vi "Teleop.vi"(10 "Match Info":T1={"Autonomous Elapsed Seconds"=0.0, "TeleOp Elapsed Seconds"=0.0, "Disabled Elapsed Seconds"=0.0, "Visited Autonomous"=FALSE, "Visited TeleOp"=FALSE, "Visited Disabled"=FALSE, "Autonomous Settings"={"Autonomous Style"=enum."Independent", "VI Refnum"=refnum}}, 11 "Call Context":T2) -> ()   [LabVIEW 2015]
doc: "This VI is called for each TeleOp packet received from the DS where the robot is not disabled. It is often used to read from the joysticks and update I/O or to update setpoints for timed control loops. It should complete and return within 20 milliseconds or it may miss DS packets."
uses:
  <vilib>/Rock Robotics/WPI/DriverStation/WPI_DriverStationDerivedRobotMode.ctl
  <vilib>/Rock Robotics/WPI/DriverStation/WPI_DriverStationMatch Info.ctl
  <vilib>/Rock Robotics/WPI/Utilities/WPI_GetSetVariantRefNum.vi
  <vilib>/Rock Robotics/Network Tables/NT Read Boolean.vi
  <vilib>/Rock Robotics/Network Tables/NT Read Number.vi
  Robot Global Data.vi
  <vilib>/Rock Robotics/Network Tables/NT Write Numeric Array.vi
panel:
  out "Sample Slider 0":dbl(slide) scale=0.0..5.0
  out "Sample Boolean 1":bool
  out "Sample Boolean 0":bool
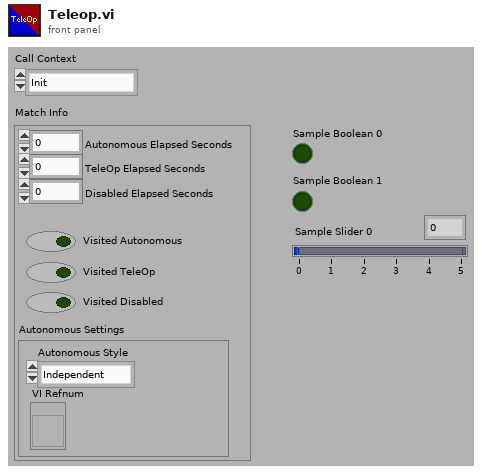
[diagram p1: front panel]
types:
  T1 = typedef "WPI_DriverStationMatch Info.ctl" = cluster{"Autonomous Elapsed Seconds":dbl, "TeleOp Elapsed Seconds":dbl, "Disabled Elapsed Seconds":dbl, "Visited Autonomous":bool, "Visited TeleOp":bool, "Visited Disabled":bool, "Autonomous Settings":cluster{"Autonomous Style":enum16{"Iterative", "Independent"}, "VI Refnum":refnum<vi>}}
  T2 = typedef "WPI_DriverStationDerivedRobotMode.ctl" = enum16{"Init", "Execute", "Stop"}
  T3 = typedef "WPI_JoystickDevRef.ctl" = cluster{"Device":T4}
  T4 = typedef "WPI_JoystickDeviceEnum.ctl" = enum16{"USB 0", "USB 1", "USB 2", "USB 3", "USB 4", "USB 5"}
  T5 = typedef "WPI_RobotDriveDevRef.ctl" = cluster{"DevStatus":errorcluster, "Motors[]":T6[], "Square Inputs":bool, "Max Output":dbl}
  T6 = typedef "WPI_MotorControlDeviceRef.ctl" = cluster{"DeviceStatus":errorcluster, "Type":T7, "PWM":cluster{"PWM Channel":T8, "DeadBand":T9}, "CAN":cluster{"Device Number":u8, "Control Mode":T10, "Semaphore":T11, "Max Vout":dbl, "TalonSRX Control Mode":T12}, "Invert":bool}
  T7 = typedef "WPI_MotorControlType.ctl" = enum16{"PWM", "CAN", "CANTalonSRX"}
  T8 = typedef "FPGA_DIOPWMChannel.ctl" = enum8{"PWM 0", "PWM 1", "PWM 2", "PWM 3", "PWM 4", "PWM 5", "PWM 6", "PWM 7", "PWM 8", "PWM 9", "PWM MXP 0", "PWM MXP 1", "PWM MXP 2", "PWM MXP 3", "PWM MXP 4", "PWM MXP 5", "PWM MXP 6", "PWM MXP 7", "PWM MXP 8", "PWM MXP 9", "Invalid"}
  T9 = typedef "WPI_PWMDeadband.ctl" = cluster{"Name":string, "maxPositivePwm":i32, "minPositivePwm":i32, "centerPwm":i32, "maxNegativePwm":i32, "minNegativePwm":i32, "angularRange":u16}
  T10 = typedef "WPI_CANJaguar_ControlMode.ctl" = enum8{"Percent VBus", "Current", "Speed", "Position", "Voltage"}
  T11 = typedef "Semaphore RefNum" = refnum<k1>
  T12 = typedef "WPI_CANTalonSRX_APIControlMode.ctl" = enum8{"Percent VBus", "Speed", "Position", "Slave", "Unchanged / Invalid", "Voltage Compensation", "Current", "Motion Profile"}
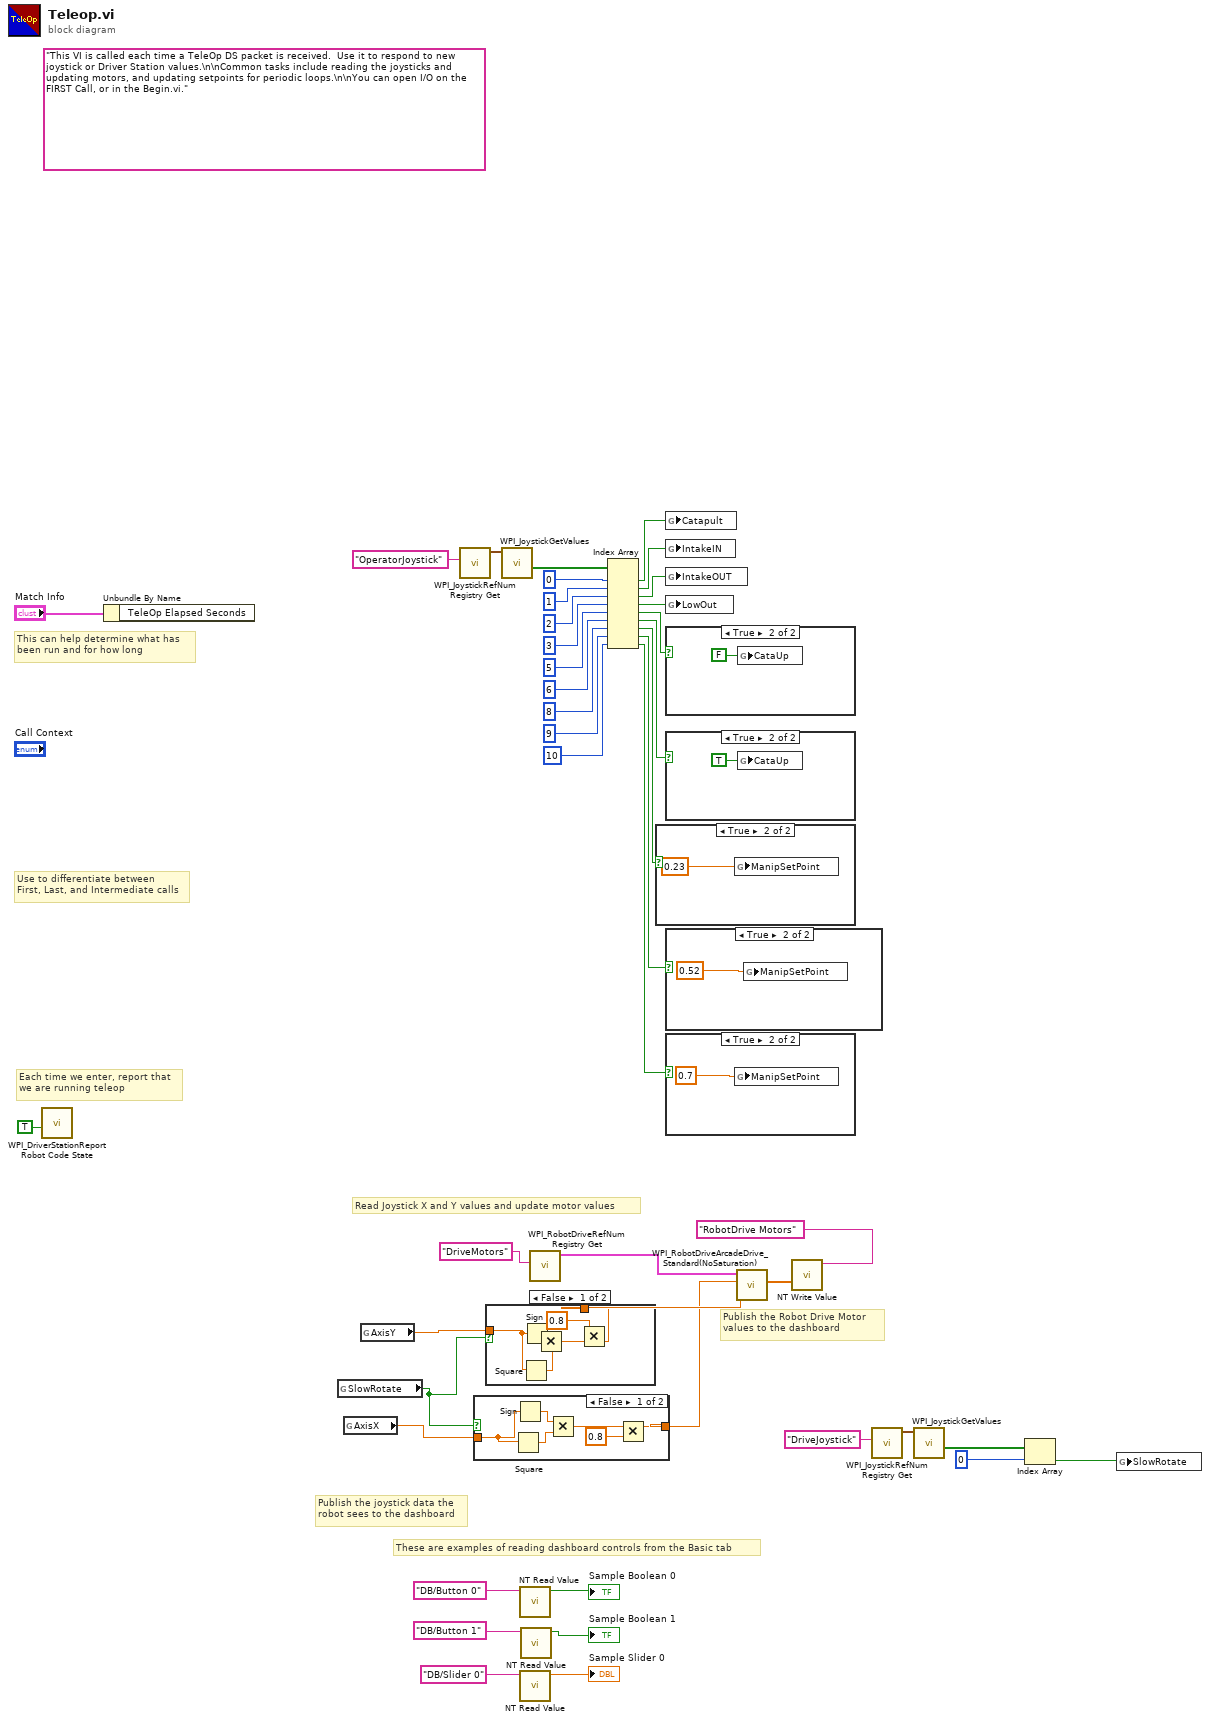
[diagram p0: block diagram]
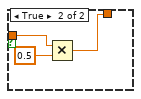
[diagram p2: hidden frame]
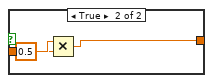
[diagram p3: hidden frame]
diagram:
  (unwired) "This VI is called each time a TeleOp DS packet is received.  Use it to respond to new joystick or Driver Station values.\n\nCommon tasks include reading the joysticks and updating motors, and updating setpoints for periodic loops.\n\nYou can open I/O on the FIRST Call, or in the Begin.vi."
  # "These are examples of reading dashboard controls from the Basic tab"
  # "Publish the Robot Drive Motor\nvalues to the dashboard"
  # "Publish the joystick data the\nrobot sees to the dashboard"
  # "Each time we enter, report that\nwe are running teleop"
  # "Use to differentiate between\nFirst, Last, and Intermediate calls"
  # "This can help determine what has\nbeen run and for how long"
  # "Read Joystick X and Y values and update motor values"
  n1 = call <vilib>:"WPI_DriverStationReport Robot Code State.vi"("TeleOp"=TRUE ("Autonomous")) -> ()  [unwired: 10 in, 1 out]
  n2 = Unbundle By Name("Match Info") -> ()  [unwired: 1 out]
  n3 = global read "Robot Global Data.vi" "SlowRotate"() -> (w3:bool)
  n4 = global read "Robot Global Data.vi" "AxisX"() -> (w19:dbl)
  n5 = global read "Robot Global Data.vi" "AxisY"() -> (w20:dbl)
  n6 = call <vilib>:"WPI_JoystickRefNum Registry Get.vi"("refnum name"="OperatorJoystick") -> ("JoystickDevRef"=w31:T3)  [unwired: 9 in, 1 out]
  n7 = case shown="False" w3 {
    tunnel: [w45 w52] -> w1
    tunnel: w19 -> [w46 w51]
    frame False {
      n8 = Square(x=w46) -> (x^2=w47:dbl)
      n9 = Sign(1:w46) -> (0:w48:dbl)
      n10 = Multiply(x=w48, y=w47) -> (x*y=w49:dbl)
      n11 = Multiply(x=w49, y=0.8) -> (x*y=w45:dbl)
    }
    frame True {
      n12 = Multiply(x=w51, y=0.5) -> (x*y=w52:dbl)
    }
  }
  n13 = case shown="False" w3 {
    tunnel: [w54 w61] -> w2
    tunnel: w20 -> [w56 w60]
    frame False {
      n14 = Square(x=w56) -> (x^2=w55:dbl)
      n15 = Sign(1:w56) -> (0:w57:dbl)
      n16 = Multiply(x=w57, y=w55) -> (x*y=w58:dbl)
      n17 = Multiply(x=0.8, y=w58) -> (x*y=w54:dbl)
    }
    frame True {
      n18 = Multiply(x=w60, y=0.5) -> (x*y=w61:dbl)
    }
  }
  n19 = call <vilib>:"WPI_JoystickGetValues.vi"("JoystickDevRef"=w31) -> ("Buttons"=w30:bool[])  [unwired: 6 in, 4 out]
  n20 = call-poly <vilib>:"NT Read Value.vi"("Name"="DB/Button 0" ("refnum name")) -> ("Boolean"=→"Sample Boolean 0":bool)  [unwired: 9 in, 1 out]
  n21 = call-poly <vilib>:"NT Read Value.vi"("Name"="DB/Slider 0" ("refnum name")) -> ("Numeric"=→"Sample Slider 0":dbl)  [unwired: 9 in, 1 out]
  n22 = call-poly <vilib>:"NT Read Value.vi"("Name"="DB/Button 1" ("refnum name")) -> ("Boolean"=→"Sample Boolean 1":bool)  [unwired: 9 in, 1 out]
  n23 = call <vilib>:"WPI_RobotDriveRefNum Registry Get.vi"("refnum name"="DriveMotors") -> ("RobotDriveDevRef"=w41:T5)  [unwired: 1 in, 9 out]
  n24 = Index Array(array=w30, index #1=0 ("index"), index #2=1 ("index"), index #3=2 ("index"), index #4=3 ("index"), index #5=5 ("index"), index #6=6 ("index"), index #7=8 ("index"), index #8=9 ("index"), index #9=10 ("index")) -> (element #1=w29:bool, element #2=w25:bool, element #3=w24:bool, element #4=w21:bool, element #5=w12:bool, element #6=w11:bool, element #7=w6:bool, element #8=w5:bool, element #9=w4:bool)
  n25 = case shown="True" w6 {
    frame False {
    }
    frame True {
      n26 = global write "Robot Global Data.vi" "ManipSetPoint"(0.23 ("ManipSetPoint")) -> ()
    }
  }
  n27 = global write "Robot Global Data.vi" "Catapult"(w29) -> ()
  n28 = global write "Robot Global Data.vi" "IntakeIN"(w25) -> ()
  n29 = global write "Robot Global Data.vi" "IntakeOUT"(w24) -> ()
  n30 = global write "Robot Global Data.vi" "LowOut"(w21) -> ()
  n31 = case shown="True" w12 {
    frame False {
    }
    frame True {
      n32 = global write "Robot Global Data.vi" "CataUp"(FALSE ("CataUp")) -> ()
    }
  }
  n33 = case shown="True" w11 {
    frame False {
    }
    frame True {
      n34 = global write "Robot Global Data.vi" "CataUp"(TRUE ("CataUp")) -> ()
    }
  }
  n35 = case shown="True" w5 {
    frame False {
    }
    frame True {
      n36 = global write "Robot Global Data.vi" "ManipSetPoint"(0.52 ("ManipSetPoint 2")) -> ()
    }
  }
  n37 = case shown="True" w4 {
    frame False {
    }
    frame True {
      n38 = global write "Robot Global Data.vi" "ManipSetPoint"(0.7 ("ManipSetPoint 3")) -> ()
    }
  }
  n39 = call <vilib>:"WPI_RobotDriveArcadeDrive_Standard(NoSaturation).vi"("Y axis value"=w2, "X axis value"=w1, "RobotDriveDevRef"=w41) -> ("Motor Values"=w33:dbl[])  [unwired: 1 in, 7 out]
  n40 = call-poly <vilib>:"NT Write Value.vi"("Numeric Array"=w33, "Name"="RobotDrive Motors") -> ()  [unwired: 9 in, 1 out]
  n41 = call <vilib>:"WPI_JoystickRefNum Registry Get.vi"("refnum name"="DriveJoystick") -> ("JoystickDevRef"=w18:T3)  [unwired: 9 in, 1 out]
  n42 = call <vilib>:"WPI_JoystickGetValues.vi"("JoystickDevRef"=w18) -> ("Buttons"=w17:bool[])  [unwired: 6 in, 4 out]
  n43 = Index Array(array=w17, index=0) -> (element=w14:bool)
  n44 = global write "Robot Global Data.vi" "SlowRotate"(w14) -> ()
